vi "Get Programs row for daily report.vi"(11 "Refnum in":T1) -> (0 "error out":errorcluster, 1 "Array out":string[][](array[string]), 2 "Numeric":i32, 3 "data Out 3":variant[][](array[variant]))   [LabVIEW 2015]
uses:
  <vilib>/addons/database/Connection.llb/Conn ObjectReference.ctl
  <userlib>/origin_lib_main/DB_Interface/DB Operations Enum.ctl
  <userlib>/_OpenG.lib/array/array.llb/Remove Duplicates from 1D Array (String)__ogtk.vi
  <userlib>/origin_lib_main/DB_Interface/DB Interface.lvlib
  <vilib>/addons/database/NI_Database_API.lvlib
panel:
  out "Array":bool[](array[boolean])
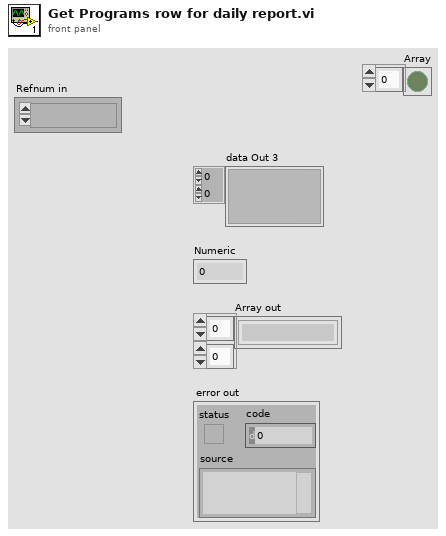
[diagram p1: front panel]
types:
  T1 = typedef "NI_Database_API.lvlib/Conn ObjectReference.ctl" = refnum<k1>
  T2 = typedef "DB Interface.lvlib/DB Operations Enum.ctl" = enum16{"Select", "Update", "Insert", "Delete", "Fetch SQL Query", "Execute SQL Query", "Drop Table", "List Tables"}
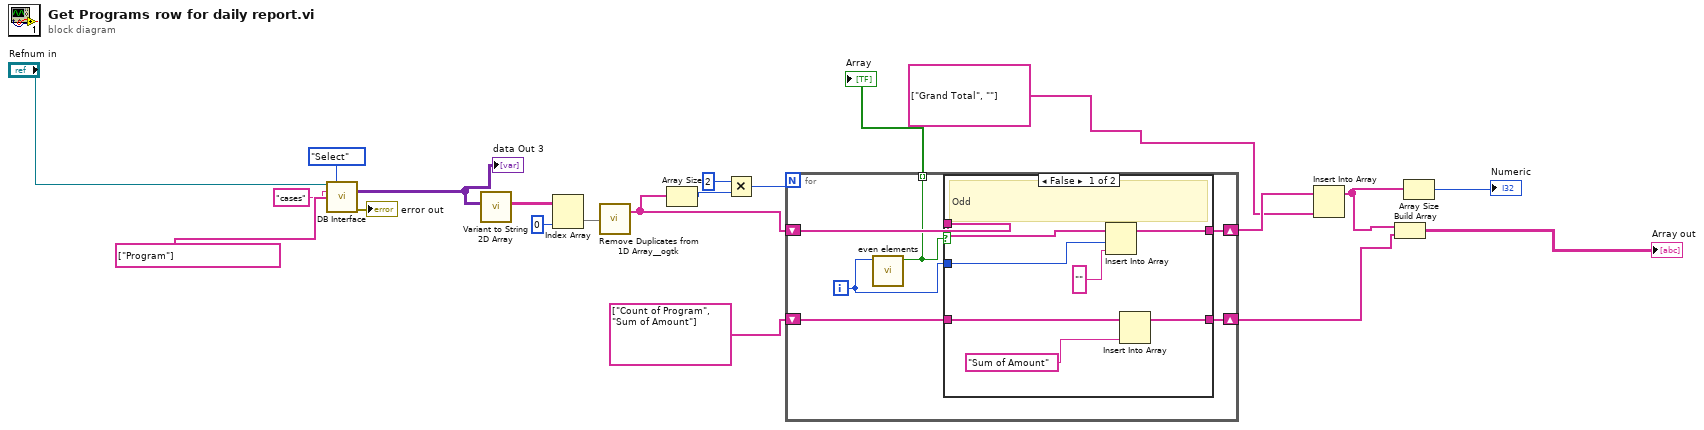
[diagram p0: block diagram]
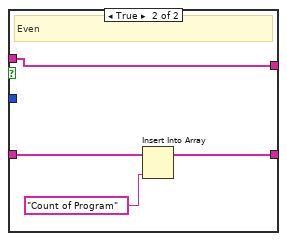
[diagram p2: hidden frame]
diagram:
  n1 = call <userlib>:"DB Interface.vi"("DB Ref In"="Refnum in", "Operation"=DB_Operations_Enum."Select", "DB Table"="cases", "DB columns"=string[] ["Program"]) -> ("data Out"=w11:variant[][], "error out"=→"error out":errorcluster)  [unwired: 8 in, 2 out]
  "data Out 3" <- w11
  n2 = call <userlib>:"Variant to String 2D Array.vi"("data Out"=w11) -> ("data"=w16:string[][])  [unwired: 9 in, 1 out]
  n3 = Index Array(array=w16, index (col)=0 ("disabled index (col)")) -> (element=w18:string[])  [unwired: 1 in]
  n4 = call-poly <userlib>:"Remove Duplicates from 1D Array__ogtk.vi"("Input Array"=w18) -> ("Output Array"=w7:string[])  [unwired: 1 out]
  n5 = Array Size(array=w7) -> (size(s)=w6:i32)
  n6 = Multiply(x=2, y=w6) -> (x*y=w5:i32)
  n7 = for {
    N: w5 -> [_]
    shift-right: [w26] -> w20
    shift-left: w7 -> [w27]
    tunnel: [w24] -> w8 mode=indexing
    shift-right: [w22] -> w2
    shift-left: string[] ["Count of Program", "Sum of Amount"] -> [w23]
    i -> [w25]
    n8 = call "even elements.vi"("Numeric"=w25) -> ("Even? (count of program)"=w24:bool)  [unwired: 10 in]
    n9 = case shown="False" w24 {
      tunnel: w27 -> [w34 w38]
      tunnel: [w32 w38] -> w26
      tunnel: w25 -> [w31 _]
      tunnel: w23 -> [w30 w36]
      tunnel: [w29 w37] -> w22
      frame False {
        # "Odd"
        n10 = Insert Into Array(array=w34, index=w31, new element="" ("new element/subarray")) -> (w32:string[])
        n11 = Insert Into Array(array=w30, new element="Sum of Amount" ("String")) -> (w29:string[])  [unwired: 1 in]
      }
      frame True {
        # "Even"
        n12 = Insert Into Array(array=w36, new element="Count of Program" ("String")) -> (w37:string[])  [unwired: 1 in]
      }
    }
  }
  "Array" <- w8
  n13 = Insert Into Array(array=w20, new element=string[] ["Grand Total", ""]) -> (w21:string[])  [unwired: 1 in]
  n14 = Build Array(w21, w2) -> (→"Array out":string[][])
  n15 = Array Size(array=w21) -> (size(s)=→"Numeric":i32)
